vi "IsUserDefinedTestVI.vi"(8 "error in (no error)":errorcluster, 11 "VI Refnum":refnum<vi>) -> (0 "error out":errorcluster, 2 "Is user-defined test VI":bool)   [LabVIEW 2019]
doc: "Returns true if the specified VI Refnum points to a user-defined test VI for the Unit Test Framework."
panel:
  out "Control Value:Get Type":variant
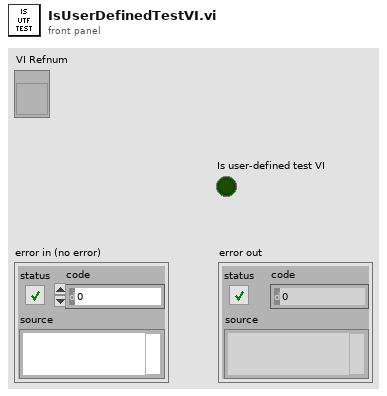
[diagram p1: front panel]
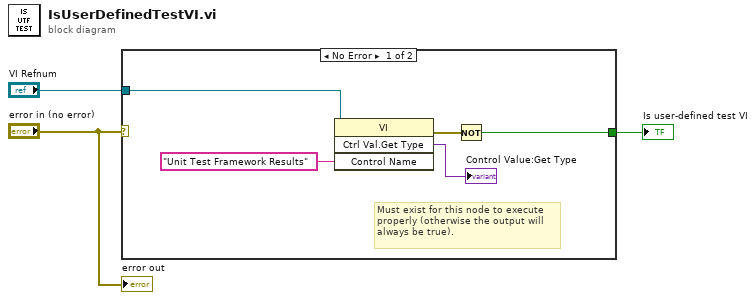
[diagram p0: block diagram]
diagram:
  n1 = case shown="No Error" "error in (no error)" {
    tunnel: "VI Refnum" -> [w8 _]
    tunnel: [w5 _] -> w2
    frame No Error {
      # "Must exist for this node to execute\nproperly (otherwise the output will\nalways be true)."
      n2 = invoke class="VI" method="Ctrl Val.Get Type"(reference=w8, "Control Name"="Unit Test Framework Results") -> (error out=w6:errorcluster, "Ctrl Val.Get Type"=→"Control Value:Get Type":variant)  [unwired: 2 in, 2 out]
      n3 = Not(x=w6) -> (.not. x?=w5:bool)
    }
    frame Error {
    }
  }
  "Is user-defined test VI" <- w2
  "error out" <- "error in (no error)"
